vi "ReplaceDatabase.vi"(6 "delimiter":string=";", 8 "Error In":errorcluster, 10 "Database path array":path[](array[path]), 11 "Selected Library URLs":string[](array[string])) -> (0 "Error Out":errorcluster)   [LabVIEW 2014]
doc: "<B>Copyright</B>: (c) MHWirth 2015. All rights reserved.\n\nThis VI gets all deployed shared variables on the given container, and finds their URL and Type. Information is written on the CSV file whose location is provided.\n\nIf the type is not defined, Status will be \"Undefined Type\", and initialization stops at the shared variable index."
panel:
  out "Name - Type":string[][](array[string])
  out "Number of Deployed SV":i32
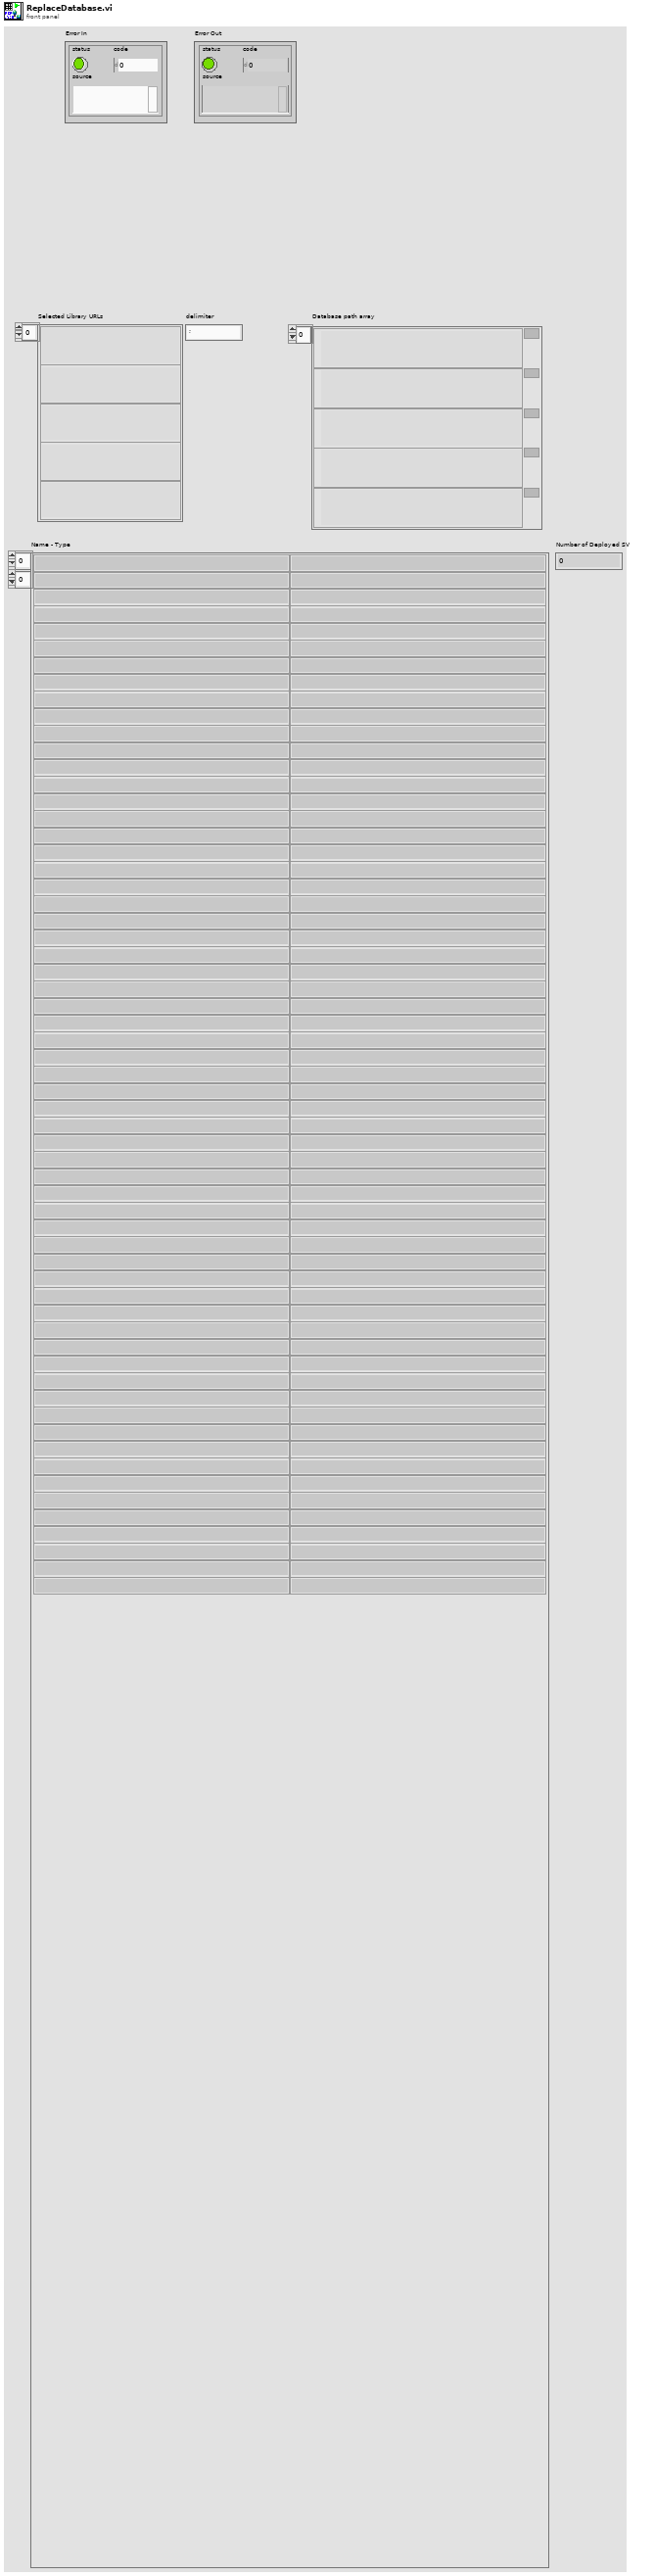
[diagram p1: front panel]
types:
  T1 = cluster{"Number of Variables":i32, "Variable/Parent Name array":string[][], "URL array":string[], "Type array":string[]}
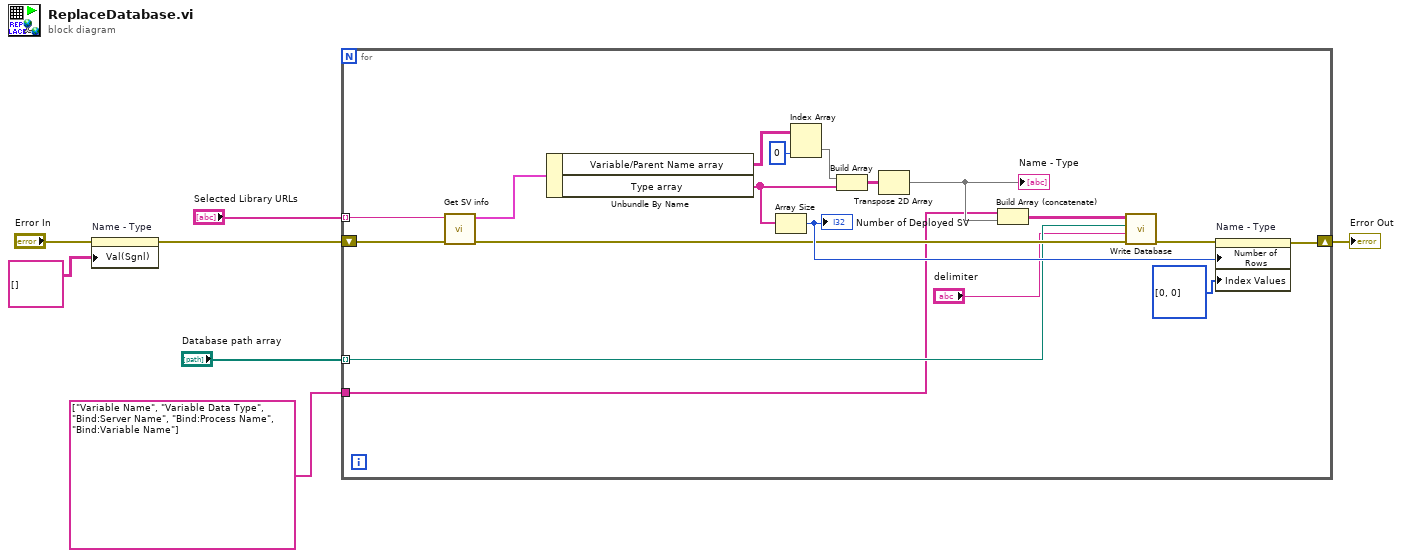
[diagram p0: block diagram]
diagram:
  n1 = property on="Name - Type" class="Arr (strict)"(error in="Error In", "Val(Sgnl)"=string[][] [] ("Value (Signaling)")) -> (error out=w2:errorcluster)  [unwired: 1 in, 1 out]
  n2 = for {
    shift-right: [w24] -> w3
    shift-left: w2 -> [w25]
    tunnel: "Database path array" -> [w12] mode=indexing
    tunnel: "Selected Library URLs" -> [w23] mode=indexing
    tunnel: string[] ["Variable Name", "Variable Data Type", "Bind:Server Name", "Bind:Process Name", "Bind:Variable Name"] -> [w9]
    n3 = call "Get SV info.vi"("Error In"=w25, "container refnum in"=w23) -> ("Error Out"=w13:errorcluster, "Deployed Shared Variable Information"=w19:T1)  [unwired: 7 in, 1 out]
    n4 = Unbundle By Name(w19) -> ("Variable/Parent Name array"=w20:string[][], "Type array"=w17:string[])
    n5 = Array Size(array=w17) -> (size(s)=w16:i32)
    "Number of Deployed SV" <- w16
    n6 = Index Array(array=w20, index (col)=0 ("disabled index (col)")) -> (element=w18:string[])  [unwired: 1 in]
    n7 = Build Array(w18, w17) -> (w22:string[][])
    n8 = Transpose 2D Array(2D array=w22) -> (transposed array=w10:string[][])
    "Name - Type" <- w10
    n9 = Build Array (concatenate)(w9, w10) -> (w8:string[][])
    n10 = call "Write Database.vi"("Error In"=w13, "delimiter (\\t)"="delimiter", "DB Path"=w12, "Data in"=w8) -> ("Error Out"=w14:errorcluster)  [unwired: 7 in]
    n11 = property on="Name - Type" class="Arr (strict)"(error in=w14, "Number of Rows"=w16, "Index Values"=u32[] [0, 0] ("Selection Start[]")) -> (error out=w24:errorcluster)  [unwired: 1 in, 1 out]
  }
  "Error Out" <- w3
